vi "Config Save.vi"(7 "Hardware Case Selection":enum16{"Init", "Read", "Write", "Close"}(ring), 8 "error in (no error)":errorcluster, 11 "Cluster":T1) -> (0 "error out":errorcluster, 3 "Data Out":T1)   [LabVIEW 2021]
uses:
  Controls/Cluster_Typedef.ctl
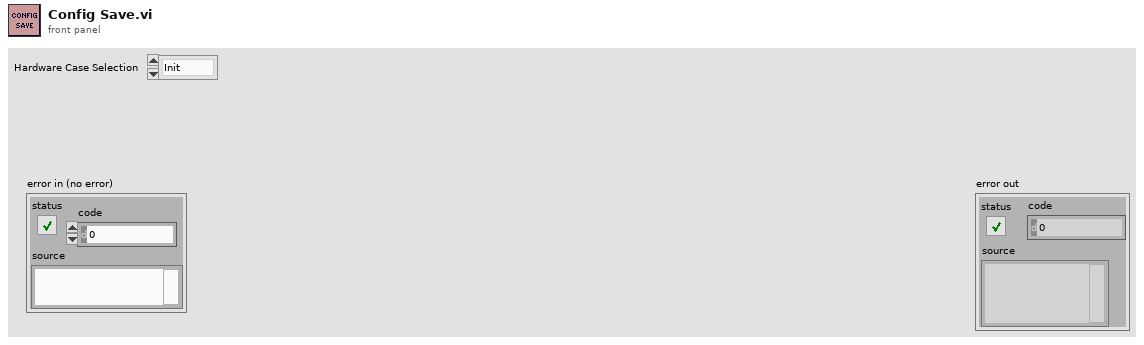
[diagram p1: front panel]
types:
  T1 = typedef "Cluster_Typedef.ctl" = cluster{"GSM":cluster{"GSM-Data":cluster{"GSM-SDR":cluster{"DL Reference Power":i32, "Serail Name":string, "UL Reference Power":i32, "Radio Device":string}, "GSM-PHY":cluster{"RACH Maximum Retransmission":string, "RACH Transmission Slots":string, "RACH Call Reestablishment":string, "RACH Access Control Class":string, "Block for Access Grant":string, "Multiframe for Paging":string, "Power Control Indicator":string, "Radio Link Timeout":string, "Cell Reselect Hysterisis":string, "Attach/Detach Allowed":string, "CCCH Combinations":string, "t3212":i64, "DTX Indicator":string, "Power Control Level":i64, "Minimum Received Signal Level":i64, "Half Rate Support":string, "Add Reselect":string}, "GSM-CELL":cluster{"SMS Enabled":string, "Eutra Operating Bands":string, "Power Offset Indicator":string, "Early Classmark Sending Control":string, "Location Area Code":i32, "CALL Enabled":string, "Loop Back Enabled":string, "GPRS Enabled":string, "SI Type 2 ter Indicator":string, "ARFCN":i64, "Frequency Format ID":i64, "Mobile Country Code":i64, "Mobile Network Code":i64, "Cell Barred Access":string, "Downlink Frequency":i32, "Uplink Frequency":i32}, "GSM-GPRS":cluster{"Priority Access THR":string, "Acess Burst Type":string, "Nack Countdown":string, "BCCH/PDCH Measurement":string, "Routing Area Code(RAC)":i32, "Network Control Order":string, "t3168":string, "t3192":string, "Alpha":string}}, "Combo":string}, "gNodeB":cluster{"Combo":string, "gNodeB-Data":cluster{"NR-SDR":cluster{"DL Reference Power":i32, "Serail Name":string, "UL Reference Power":i32, "DL Antennas":string, "UL Antennas":string, "Radio Device":string}, "NR-PHY":cluster{"PDSCH Reference Power":i64, "SSB RSRP Threshold":i64, "PRACH Contention Resolution Timer":i64, "Preamble Per SSB":i64, "Preamble Per SSB Format":i64, "UE Power Level Grant":i64, "RA Response Window":string, "Power Ramp Step Size":string, "Preamble Root Sequence Index":string, "Preamble Transmission Count":string, "Preamble Received Power":i64, "Zero Correlation Zone Configuration":i64, "Msg Frequency Division Multiplexing":string, "PRACH Configuration Index":i64, "Preamble Timing Offset":i64, "Preamble Format":i64, "Resource Restriction Type":string}, "NR-CELL":cluster{"Tracking Area Code":i64, "Mobile Country Code":i64, "Mobile Network Code":i64, "Operating Bands":string, "Physical Cell ID":i64, "DL Offset to Carrier":i32, "Subcarrier Spacing":string, "UL Offset to Carrier 2":i32, "Carrier Bandwidth":string, "Transmission Mode":string, "CSI-RS":string, "SRS":string, "Measurement Report":string}, "NR-RRC":cluster{"Ciphering Algorithms for SRB":string, "Integrity Algorithms for SRB":string, "Ciphering Algorithms for DRB":string, "Integrity Algorithms for DRB":string}}}, "eNodeB":cluster{"Combo":string, "eNodeB-Data":cluster{"LTE-SDR":cluster{"Radio Device":string, "DL Reference Power":i32, "Serail Name":string, "UL Reference Power":i32, "DL Antennas":string, "UL Antennas":string}, "LTE-PHY":cluster{"PBCH Repetition":string, "PUCCH Delta Shift":string, "PUCCH CQI Number of RB":string, "PHICH Resource":string, "SRS Enable":string, "PCCH Paging Cycle":string, "BCCH Modification Coefficient":string, "PUSCH Alpha":string, "PUSCH DMRS Enable":string, "PHICH Duration":string, "PUCCH HARQ Max Transmission":i64, "PCCH Narrowband Count":string, "PUSCH Power Offset":i64, "PUCCH Power Offset":i64, "PDSCH Power Boost":string, "PUCCH An Occassions":string, "PUUCH CS Antenna Ports":string, "PRACH Response Window Size":string, "PRACH Contention Resolution Timer":string, "PRACH Ramping Step Size":string, "PDSCH Reference Power":i64, "PRACH Root Sequence Index":i64, "PRACH Maximum Transmissions":string, "PRACH Initial Received Target Power":string, "PRACH Configuration Index":i64}, "LTE-CELL":cluster{"Duplex Mode":string, "Measurement Report":string, "Eutra Operating Bands":string, "Carrier Bandwidth":string, "Physical Cell ID":i64, "Network Name":string, "DL Frequency":i32, "UL Frequency":i32, "Transmission Mode":string, "MNC Length":string, "IMS Enabled":string, "Tracking Area Code":i32, "Mobile Network Code":i32, "Mobile Country Code":i32}, "LTE-RRC":cluster{"RLC Maximum Retransmision Threshold":string, "RLC Timer Poll Retransmit":i32, "RLC Timer Reordering":i32, "RLC Timer Status Prohibit":i32, "RLC Poll PDU":i32, "RLC Poll Byte":i32}}}}
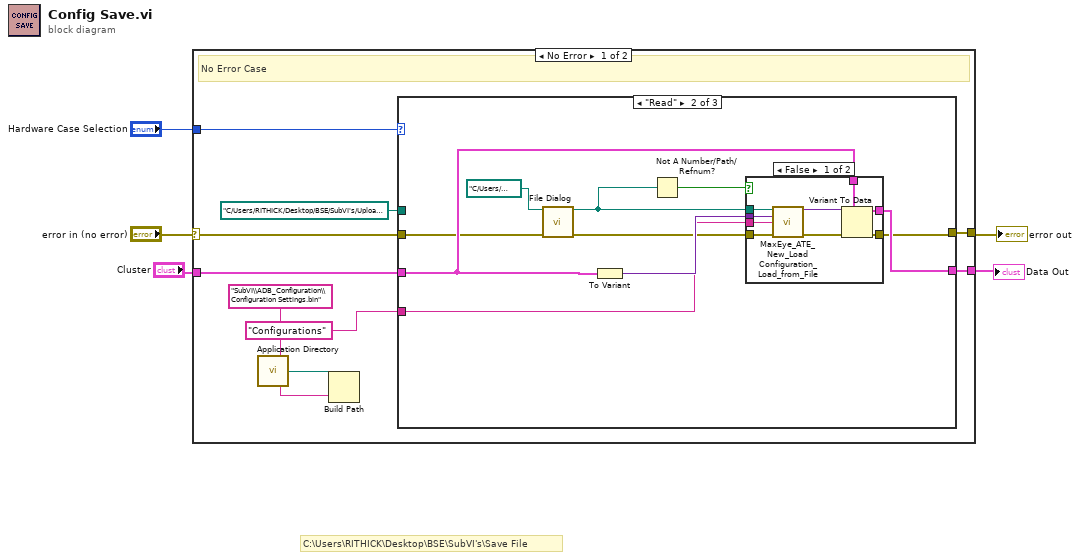
[diagram p0: block diagram]
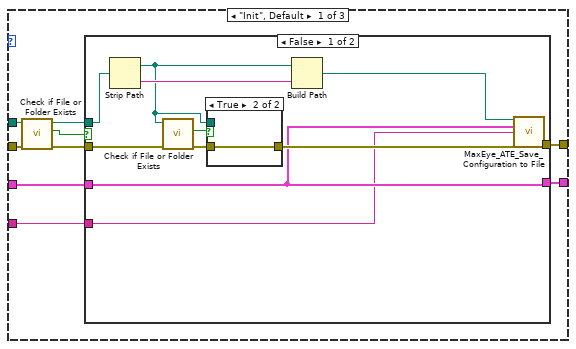
[diagram p2: hidden frame]
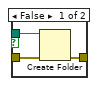
[diagram p3: hidden frame]
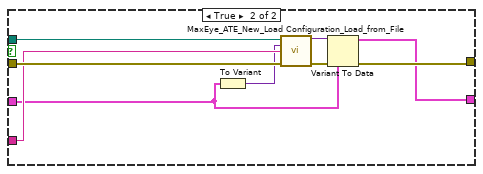
[diagram p4: hidden frame]
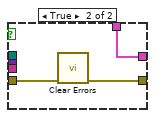
[diagram p5: hidden frame]
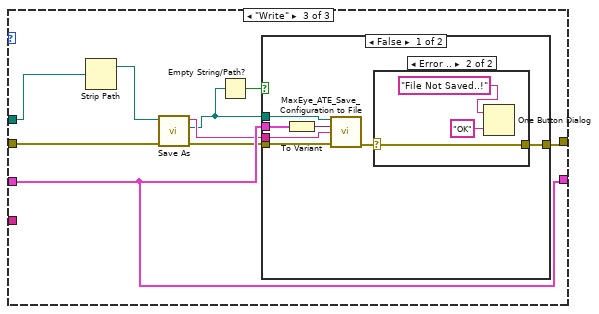
[diagram p6: hidden frame]
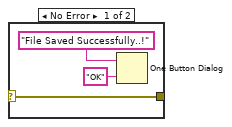
[diagram p7: hidden frame]
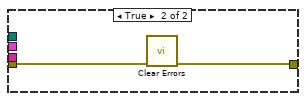
[diagram p8: hidden frame]
diagram:
  # "C:\\Users\\RITHICK\\Desktop\\BSE\\SubVI's\\Save File"
  n1 = case shown="No Error" "error in (no error)" {
    selector: "error in (no error)" -> [w12 w95]
    tunnel: [w11 w95] -> w5
    tunnel: [w10 w94] -> w1
    tunnel: "Hardware Case Selection" -> [w9 _]
    tunnel: "Cluster" -> [w8 w94]
    frame No Error {
      # "No Error Case"
      n2 = call <vilib>:"Application Directory.vi"() -> ("Application Directory"=w14:path)
      n3 = Build Path(base path=w14, name or relative path="SubVI\\ADB_Configuration\\Configuration Settings.bin") -> ()  [unwired: 1 out]
      n4 = case shown="\"Read\"" w9 {
        tunnel: path "C:/Users/RITHICK/Desktop/BSE/SubVI's/Upload & Download/Save Config/Configuration.bin" ("appended path") -> [w23 _ w74]
        tunnel: w12 -> [w22 w52 w76]
        tunnel: [w20 w55 w78] -> w11
        tunnel: [w19 w56 w77] -> w10
        tunnel: w8 -> [w17 w57 w77]
        tunnel: "Configurations" ("Config Header") -> [w16 w53 _]
        frame "Init", Default {
          n5 = call <vilib>:"Check if File or Folder Exists.vi"("error in (no error)"=w22, "path"=w23) -> ("error out"=w21:errorcluster, "file or folder exists?"=w18:bool, "dup path"=w15:path)  [unwired: 7 in]
          n6 = case shown="False" w18 {
            tunnel: w21 -> [w33 w43]
            tunnel: w15 -> [w24 w41]
            tunnel: [w28 w47] -> w20
            tunnel: [w26 w46] -> w19
            tunnel: w17 -> [w26 w39]
            tunnel: w16 -> [w25 w42]
            frame False {
              n7 = Strip Path(path=w24) -> (stripped path=w30:path, name=w34:string)
              n8 = call <vilib>:"Check if File or Folder Exists.vi"("error in (no error)"=w33, "path"=w30) -> ("error out"=w32:errorcluster, "file or folder exists?"=w31:bool)  [unwired: 7 in, 1 out]
              n9 = case shown="True" w31 {
                tunnel: w32 -> [w37 w38]
                tunnel: w30 -> [w36 _]
                tunnel: [w35 w38] -> w29
                frame False {
                  n10 = Create Folder(path (use dialog)=w36, error in=w37) -> (error out=w35:errorcluster)  [unwired: 1 in, 2 out]
                }
                frame True {
                }
              }
              n11 = Build Path(base path=w30, name or relative path=w34) -> (appended path=w27:path)
              n12 = call "MaxEye_ATE_Save_Configuration to File.vi"("file path (use dialog)"=w27, "Variant"=w26, "Config Header"=w25, "error in (no error)"=w29) -> ("error out"=w28:errorcluster)  [unwired: 11 in]
            }
            frame True {
              n13 = To Variant(anything=w39) -> (Variant=w40:variant)
              n14 = call "MaxEye_ATE_New_Load Configuration_Load_from_File.vi"("file path (use dialog)"=w41, "Variant In"=w40, "Config Header"=w42, "error in (no error)"=w43) -> ("Variant Out"=w45:variant, "error out"=w44:errorcluster)  [unwired: 10 in]
              n15 = Variant To Data(error in=w44, type=w39, Variant=w45) -> (data=w46:T1, error out=w47:errorcluster)
            }
          }
        }
        frame "Read" {
          n16 = call "File Dialog"("start path"=path "C:/Users/RITHICK/Desktop/BSE/SubVI's/Upload & Download/Save Config" ("appended path"), "error in"=w52) -> ("selected path"=w49:path, "error out"=w51:errorcluster)  [unwired: 10 in, 2 out]
          n17 = To Variant(anything=w57) -> (Variant=w54:variant)
          n18 = Not A Number/Path/Refnum?(number/path/refnum=w49) -> (NaN/Path/Refnum?=w48:bool)
          n19 = case shown="False" w48 {
            tunnel: w57 -> [w66 w69]
            tunnel: [w65 w69] -> w56
            tunnel: [w64 w67] -> w55
            tunnel: w54 -> [w63 _]
            tunnel: w53 -> [w62 _]
            tunnel: w51 -> [w59 w68]
            tunnel: w49 -> [w58 _]
            frame False {
              n20 = call "MaxEye_ATE_New_Load Configuration_Load_from_File.vi"("file path (use dialog)"=w58, "Variant In"=w63, "Config Header"=w62, "error in (no error)"=w59) -> ("Variant Out"=w61:variant, "error out"=w60:errorcluster)  [unwired: 10 in]
              n21 = Variant To Data(error in=w60, type=w66, Variant=w61) -> (data=w65:T1, error out=w64:errorcluster)
            }
            frame True {
              n22 = call <vilib>:"Clear Errors.vi"("error in (no error)"=w68) -> ("error out"=w67:errorcluster)  [unwired: 5 in, 1 out]
            }
          }
        }
        frame "Write" {
          n23 = Strip Path(path=w74) -> (stripped path=w72:path)  [unwired: 1 out]
          n24 = call "Save As.vi"("error in (no error)"=w76, "path"=w72) -> ("error out"=w75:errorcluster, "File Path"=w70:path, "File Name"=w73:string)  [unwired: 7 in]
          n25 = Empty String/Path?(string/path=w70) -> (empty?=w71:bool)
          n26 = case shown="False" w71 {
            tunnel: [w79 w92] -> w78
            tunnel: w77 -> [w84 _]
            tunnel: w75 -> [w83 w93]
            tunnel: w73 -> [w82 _]
            tunnel: w70 -> [w81 _]
            frame False {
              n27 = To Variant(anything=w84) -> (Variant=w85:variant)
              n28 = call "MaxEye_ATE_Save_Configuration to File.vi"("file path (use dialog)"=w81, "Variant"=w85, "Config Header"=w82, "error in (no error)"=w83) -> ("error out"=w80:errorcluster)  [unwired: 11 in]
              n29 = case shown="Error .." w80 {
                selector: w80 -> [w86 w89]
                tunnel: [w86 w89] -> w79
                frame No Error {
                  n30 = One Button Dialog(message="File Saved Successfully..!", button name ("OK")="OK") -> ()  [unwired: 1 out]
                }
                frame Error {
                  n31 = One Button Dialog(message="File Not Saved..!", button name ("OK")="OK") -> ()  [unwired: 1 out]
                }
              }
            }
            frame True {
              n32 = call <vilib>:"Clear Errors.vi"("error in (no error)"=w93) -> ("error out"=w92:errorcluster)  [unwired: 5 in, 1 out]
            }
          }
        }
      }
    }
    frame Error {
      # "Error case"
    }
  }
  "error out" <- w5
  "Data Out" <- w1
